vi "Color to Gradient.vi"(9 "Color Box":u32(colorbox)=10551263) -> (0 "Total Possible Gradients with Specified Color":u8, 3 "Color Gradient":u32[](array[colorbox]))   [LabVIEW 2026]
doc: "Calculates and outputs a contrast gradient of an input color from its brightest to its darkest. The output is an array of colors. This is useful if you want a darker or lighter version of an input color - that is the same color, but lighter or darker shade. As the total gradients is limited to 0 - 255 for R, G or B, the total possible gradients output for a particular color differ on how close or far any of the starting RGB values are from 0 to 255."
panel:
  # "0-255 Values"
  # "0-1 values"
  # "Overview: Takes an input color and outputs all possible light to dark shades as a color array.\nRequirements: LabVIEW 2016 or compatible\nInstructions:\n1. Specify a color value in the Color Box.\n2. Run the VI. The Color Gradient array will display the full gradient generated for the specified color, and the Animation image will display each color in the array from light to dark."
  # "``"
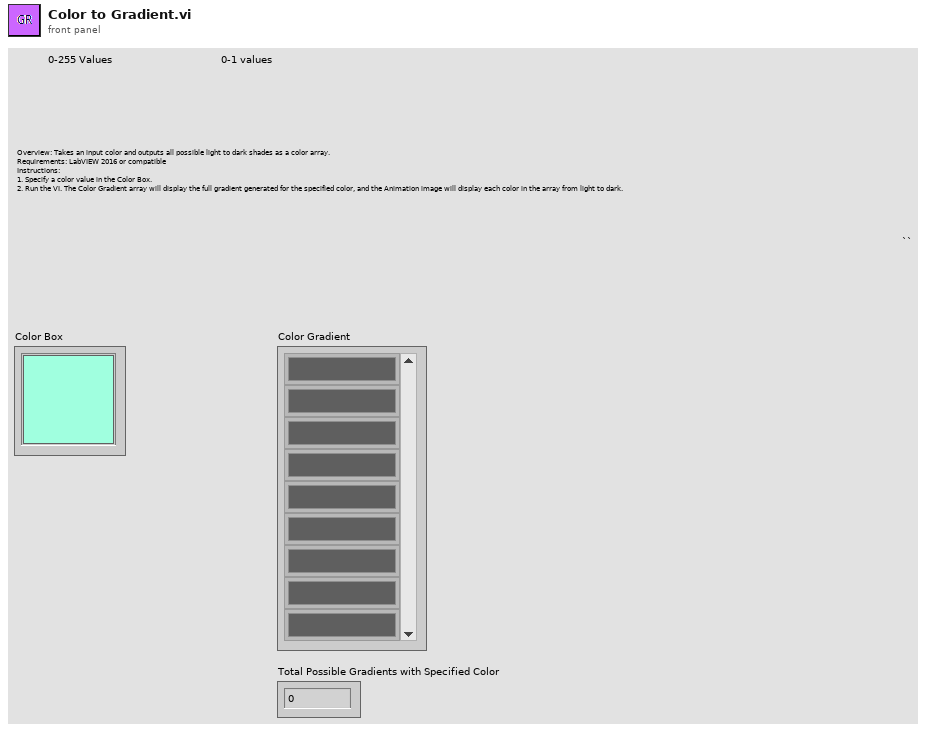
[diagram p1: front panel]
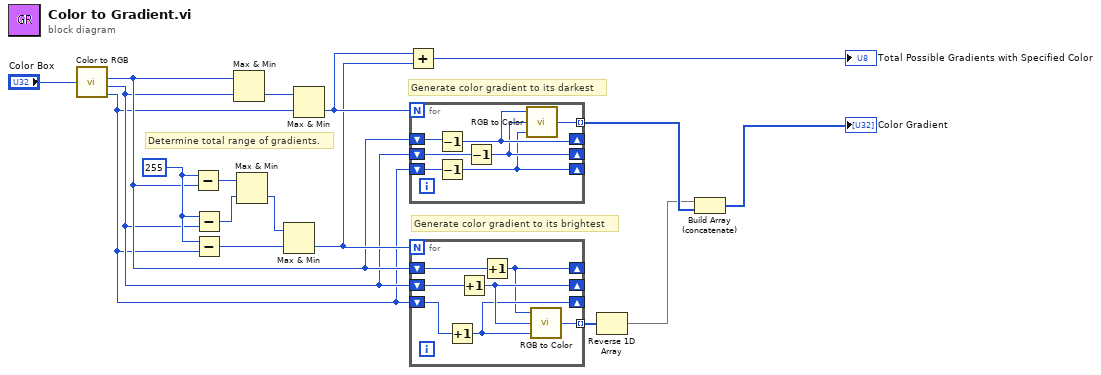
[diagram p0: block diagram]
diagram:
  w13 = u8 255
  # "Determine total range of gradients."
  # "Generate color gradient to its brightest"
  # "Generate color gradient to its darkest"
  n1 = call <vilib>:"Color to RGB.vi"("Color"="Color Box") -> ("R"=w4:u8, "G"=w3:u8, "B"=w2:u8)  [unwired: 1 out]
  n2 = Subtract(x=w13, y=w4) -> (x-y=w17:u8)
  n3 = Subtract(x=w13, y=w3) -> (x-y=w16:u8)
  n4 = Subtract(x=w13, y=w2) -> (x-y=w14:u8)
  n5 = Max & Min(x=w4, y=w3) -> (min(x,y)=w12:u8)  [unwired: 1 out]
  n6 = Max & Min(x=w17, y=w16) -> (min(x,y)=w15:u8)  [unwired: 1 out]
  n7 = Max & Min(x=w15, y=w14) -> (min(x,y)=w10:u8)  [unwired: 1 out]
  n8 = Max & Min(x=w12, y=w2) -> (min(x,y)=w11:u8)  [unwired: 1 out]
  n9 = Add(x=w11, y=w10) -> (x+y=→"Total Possible Gradients with Specified Color":u8)
  n10 = for {
    N: w11 -> [_]
    shift-right: [w21] -> _
    shift-left: w4 -> [w23]
    shift-right: [w20] -> _
    shift-left: w3 -> [w22]
    shift-right: [w19] -> _
    shift-left: w2 -> [w24]
    tunnel: [w18] -> w7 mode=indexing
    n11 = Decrement(x=w23) -> (x-1=w21:u8)
    n12 = Decrement(x=w24) -> (x-1=w19:u8)
    n13 = Decrement(x=w22) -> (x-1=w20:u8)
    n14 = call <vilib>:"RGB to Color.vi"("B"=w19, "G"=w20, "R"=w21) -> ("Color"=w18:u32)
  }
  n15 = for {
    N: w10 -> [_]
    tunnel: [w31] -> w8 mode=indexing
    shift-right: [w25] -> _
    shift-left: w4 -> [w26]
    shift-right: [w28] -> _
    shift-left: w3 -> [w29]
    shift-right: [w27] -> _
    shift-left: w2 -> [w30]
    n16 = Increment(x=w30) -> (x+1=w27:u8)
    n17 = Increment(x=w29) -> (x+1=w28:u8)
    n18 = Increment(x=w26) -> (x+1=w25:u8)
    n19 = call <vilib>:"RGB to Color.vi"("B"=w27, "G"=w28, "R"=w25) -> ("Color"=w31:u32)
  }
  n20 = Reverse 1D Array(array=w8) -> (reversed array=w6:u32[])
  n21 = Build Array (concatenate)(w6, w7) -> (→"Color Gradient":u32[])
